vi "Vision Research Phantom Series Reset.vi"(11 "Error In (no error)":errorcluster) -> (15 "Error Out":errorcluster)   [LabVIEW 2013, in "VRI.lvlib"]
doc: "This VI resets the Vision Research Phantom Series camera and then sends a set of default setup commands to the camera.\n\nWritten by:\nBLOOMY CONTROLS, INC\nWINDSOR, CT 06095, USA\n860-298-9925\nwww.bloomy.com\nV1.0.0\nMay, 2004"
uses:
  VRI.lvlib
panel:
  # "For instructions on the use of this VI, press Ctrl+H to display the help window and move the mouse over the icon, controls, and indicators"
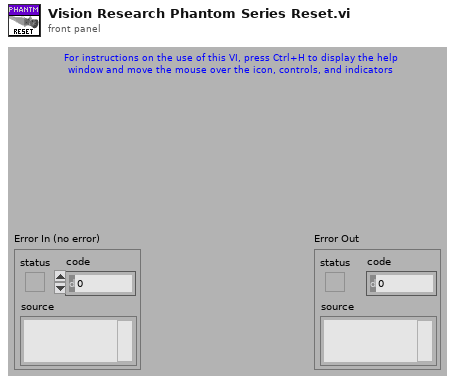
[diagram p1: front panel]
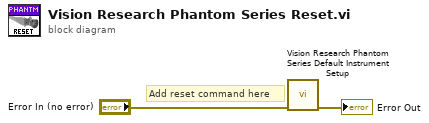
[diagram p0: block diagram]
diagram:
  # "Add reset command here"
  n1 = call "Vision Research Phantom Series Default Instrument Setup.vi"("Error In (no error)"="Error In (no error)") -> ("Error Out"=→"Error Out":errorcluster)  [unwired: 14 out]
